vi "Op-Stress-Accumulate.vi"(8 "error in (no error)":errorcluster, 9 "operation (query:0)":u16(ring) items=["query", "reset", "set to value ->"], 10 "new value":dbl format="%^.6e", 11 "VISA session":refnum<visa-resource-name>) -> (0 "error out":errorcluster, 1 "current value":dbl format="%^.4e", 3 "VISA resource name out":refnum<visa-resource-name>)   [LabVIEW 2016, in "Agilent 415X Series.lvlib"]
doc: "This VI monitors or sets the accumulated stress parameter."
uses:
  Agilent 415X Series.lvlib
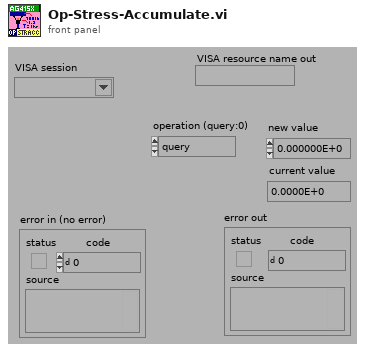
[diagram p1: front panel]
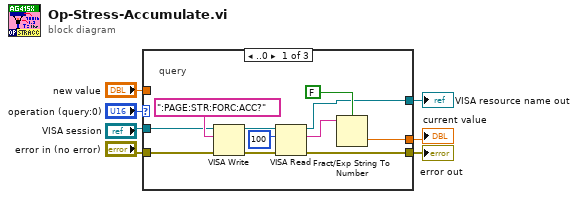
[diagram p0: block diagram]
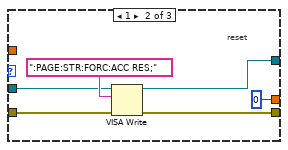
[diagram p2: hidden frame]
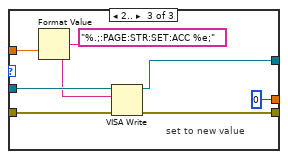
[diagram p3: hidden frame]
diagram:
  n1 = case shown="..0" "operation (query:0)" {
    tunnel: "error in (no error)" -> [w15 w23 w32]
    tunnel: "VISA session" -> [w14 w22 w31]
    tunnel: [w13 0 0] -> w3
    tunnel: [w12 w21 w30] -> w4
    tunnel: "new value" -> [_ _ w26]
    tunnel: [w8 w19 w25] -> w1
    frame ..0 {
      # "query"
      n2 = VISA Write(VISA resource name=w14, write buffer=":PAGE:STR:FORC:ACC?", error in (no error)=w15) -> (VISA resource name out=w17:refnum<visa-resource-name>, error out=w18:errorcluster)  [unwired: 1 out]
      n3 = VISA Read(VISA resource name=w17, byte count=u32 100, error in (no error)=w18) -> (VISA resource name out=w8:refnum<visa-resource-name>, read buffer=w10:string, error out=w12:errorcluster)  [unwired: 1 out]
      n4 = Fract/Exp String To Number(use system decimal point (T)=FALSE, string=w10) -> (number=w13:dbl)  [unwired: 2 in, 1 out]
    }
    frame 1 {
      # "reset"
      n5 = VISA Write(VISA resource name=w22, write buffer=":PAGE:STR:FORC:ACC RES;", error in (no error)=w23) -> (VISA resource name out=w19:refnum<visa-resource-name>, error out=w21:errorcluster)  [unwired: 1 out]
    }
    frame 2.. {
      # "set to new value"
      n6 = Format Value(format string="%.;:PAGE:STR:SET:ACC %e;", value (0)=w26) -> (output string=w27:string)  [unwired: 1 in]
      n7 = VISA Write(VISA resource name=w31, write buffer=w27, error in (no error)=w32) -> (VISA resource name out=w25:refnum<visa-resource-name>, error out=w30:errorcluster)  [unwired: 1 out]
    }
  }
  "error out" <- w4
  "current value" <- w3
  "VISA resource name out" <- w1
